vi "MMC_setDevice.vi"(3 "Error in":errorcluster, 5 "Device Number (1..16)":u8=1) -> (0 "Error out":errorcluster, 2 "function return":i32)   [LabVIEW 2024]
doc: "This vi sends the address code of the specified device. It is not verified whether the device is actually connected tothe network. Use this vi to re-address a device that was reset due to power off or other reasons."
uses:
  MMC.dll
panel:
  out "Message":string
  # "MMC_setDevice"
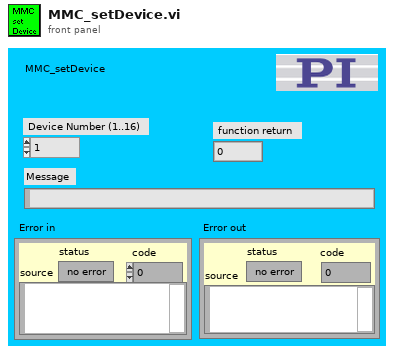
[diagram p1: front panel]
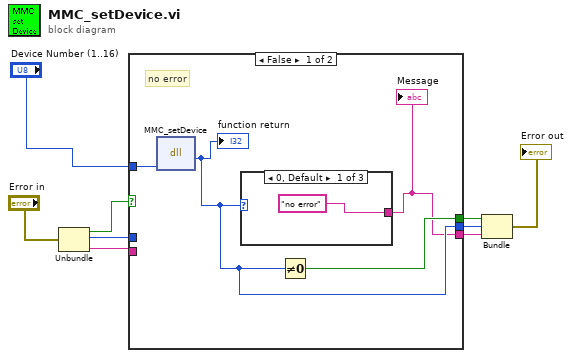
[diagram p0: block diagram]
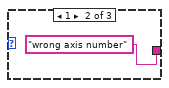
[diagram p2: hidden frame]
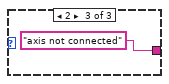
[diagram p3: hidden frame]
diagram:
  n1 = Unbundle("Error in") -> ("status"=w8:bool, "code"=w2:i32, "source"=w1:string)
  n2 = case shown="False" w8 {
    selector: w8 -> [_ w19]
    tunnel: "Device Number (1..16)" -> [w13 _]
    tunnel: [w12 w19] -> w5
    tunnel: [w10 w17] -> w4
    tunnel: [w11 w18] -> w3
    tunnel: w2 -> [_ w18]
    tunnel: w1 -> [_ w17]
    frame False {
      # "no error"
      n3 = dll-call lib="E:/Wilson/HoppingSICM_TK/HoppingSICM_v1/DLLs/MMC.dll" fn="MMC_setDevice"("newAxis"=w13) -> (w11:i32)  [unwired: 4 in, 2 out]
      "function return" <- w11
      n4 = case shown="0, Default" w11 {
        tunnel: ["no error" "wrong axis number" "axis not connected"] -> w10
        frame 0, Default {
        }
        frame 1 {
        }
        frame 2 {
        }
      }
      "Message" <- w10
      n5 = Not Equal To 0?(x=w11) -> (x != 0?=w12:bool)
    }
    frame True {
      # "error"
    }
  }
  n6 = Bundle(w5, "code"=w3, "source"=w4) -> (→"Error out":cluster{bool, "code":i32, "source":string})  [unwired: 1 in]
